vi "Source Offset.vi"(8 "error in (no error)":errorcluster, 10 "Mode":u16(ring) items=["GET", "OFF"], 11 "VISA resource name":refnum<visa-resource-name>) -> (0 "error out":errorcluster, 3 "VISA resource name out":refnum<visa-resource-name>)   [LabVIEW 2025, in "Chroma 19572.lvlib"]
doc: "Chroma\n5 Clock Tower Place Suite 210\nMaynard, MA 01754\nTel: 1 800 253-1230\nTel: 1 877 4 A HIPOT\nFax: 1 978-461-4295\nWebsite: www.chroma.com"
uses:
  <instrlib>/Chroma 19572/Chroma 19572.lvlib
panel:
  # "GET: Run OFFSET measure for AC & DC modes only\nOFF: Turn off OFST label on Instrument Display"
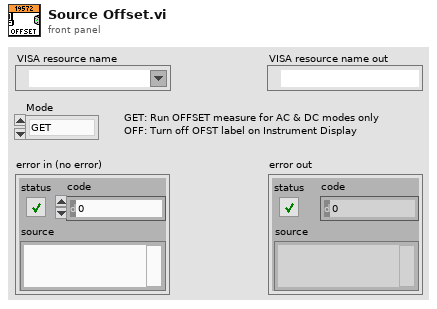
[diagram p1: front panel]
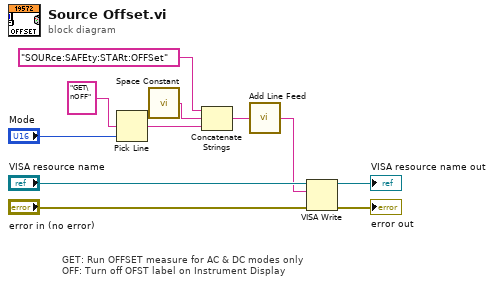
[diagram p0: block diagram]
diagram:
  # "GET: Run OFFSET measure for AC & DC modes only\nOFF: Turn off OFST label on Instrument Display"
  n1 = Pick Line(multi-line string="GET\nOFF", line index="Mode") -> (output string=w3:string)  [unwired: 1 in]
  n2 = call <vilib>:"Space Constant.vi"() -> ("String"=w4:string)
  n3 = Concatenate Strings("SOURce:SAFEty:STARt:OFFSet", w4, w3) -> (w1:string)
  n4 = call <instrlib>:"Add Line Feed.vi"("Command string"=w1) -> ("Concatenated string"=w2:string)  [unwired: 4 in]
  n5 = VISA Write(VISA resource name="VISA resource name", write buffer=w2, error in (no error)="error in (no error)") -> (VISA resource name out=→"VISA resource name out":refnum<visa-resource-name>, error out=→"error out":errorcluster)  [unwired: 1 out]
